vi "Configure Source Function.vi"(8 "error in (no error)":errorcluster, 10 "Function (0: Volts)":u16(ring) items=["Volts", "Current"], 11 "VISA resource name":refnum<visa-resource-name>) -> (0 "error out":errorcluster, 3 "VISA resource name out":refnum<visa-resource-name>)   [LabVIEW 2015, in "Keithley 2450.lvlib"]
doc: "Configures the source function on the instrument."
uses:
  <instrlib>/Keithley 2450/Keithley 2450.lvlib
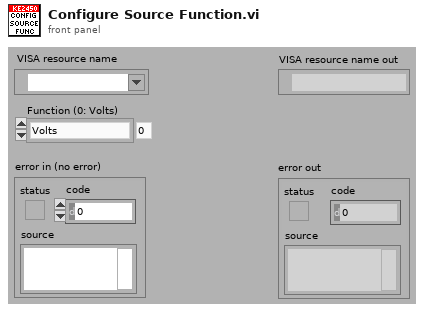
[diagram p1: front panel]
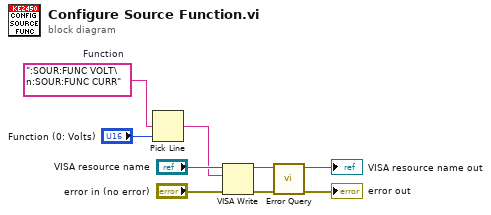
[diagram p0: block diagram]
diagram:
  w5 = ":SOUR:FUNC VOLT\n:SOUR:FUNC CURR"  # Function
  n1 = Pick Line(multi-line string=w5, line index="Function (0: Volts)") -> (output string=w1:string)  [unwired: 1 out]
  n2 = VISA Write(VISA resource name="VISA resource name", write buffer=w1, error in (no error)="error in (no error)") -> (VISA resource name out=w3:refnum<visa-resource-name>, error out=w2:errorcluster)  [unwired: 1 out]
  n3 = call <instrlib>:"Error Query.vi"("error in (no error)"=w2, "VISA resource name"=w3) -> ("error out"=→"error out":errorcluster, "VISA resource name out"=→"VISA resource name out":refnum<visa-resource-name>)  [unwired: 8 out]
